vi "vControl_e.vi"(2 "v Ctrl in":refnum<class "CtrlLine.lvclass">[](array[class]), 7 "QuWire in":refnum<class "QuWire.lvclass">) -> (8 "QuWire out":refnum<class "QuWire.lvclass">, 13 "v Ctrl out":refnum<class "CtrlLine.lvclass">)   [LabVIEW 2020]
doc: "Control Node\n\nCondition for a Controlled Operation. \nThe target gate is applied ONLY if this control qubit is in the |1> state.\n\nBlock Matrix Structure: [[ 1, 0], [ 0, U]] Where U is the target operation."
uses:
  QuSim/QuWire/QuWire.lvclass
  QuSim/QuWire/CtrlLine/CtrlLine.lvclass
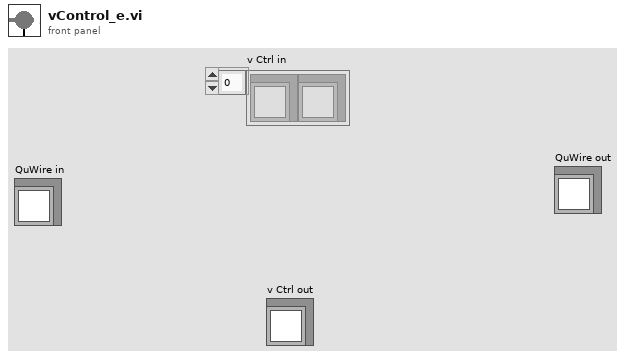
[diagram p1: front panel]
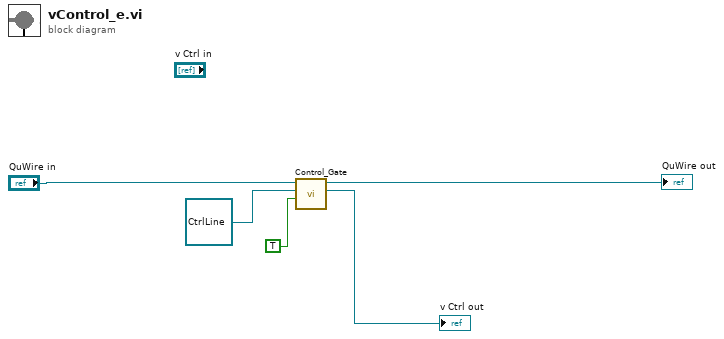
[diagram p0: block diagram]
diagram:
  n1 = call "Control_Gate.vi"("Control/Anti-control ?"=TRUE, "CtrlLine in"=refnum<class "CtrlLine.lvclass"> refnum ("u Ctrl Line in"), "QuWire in"="QuWire in") -> ("CtrlLine out"=→"v Ctrl out":refnum<class "CtrlLine.lvclass">, "QuWire out"=→"QuWire out":refnum<class "QuWire.lvclass">)  [unwired: 6 in, 1 out]
